vi "ThisLevelClassName.vi"(11 "SMO":refnum<class "SMO.lvclass">) -> (2 "Level class name":string, 3 "SMO out":refnum<class "SMO.lvclass">)   [LabVIEW 2021, in "smo.lvlib" / "SMO.lvclass"]
uses:
  SMO.lvclass
  SMO.lvclass/SMO.ctl
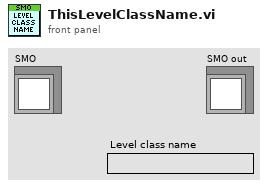
[diagram p1: front panel]
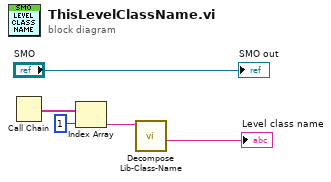
[diagram p0: block diagram]
diagram:
  n1 = Call Chain() -> (call chain=w5:string[])
  n2 = Index Array(array=w5, index=1) -> (element=w2:string)
  n3 = call "Decompose Lib-Class-Name.vi"("Qualified Name"=w2) -> ("className"=→"Level class name":string)  [unwired: 6 in, 4 out]
  "SMO out" <- "SMO"
